vi "初始化.vi"(8 "error in (no error)":errorcluster caption="错误输入（无错误）", 11 "堆栈 输入":refnum<class "堆栈(STR).lvclass"> caption="DNL_LabVIEW Object in") -> (0 "error out":errorcluster caption="错误输出", 3 "堆栈输出":refnum<class "堆栈(STR).lvclass"> caption="DNL_LabVIEW Object out")   [LabVIEW 2012, in "堆栈(STR).lvclass"]
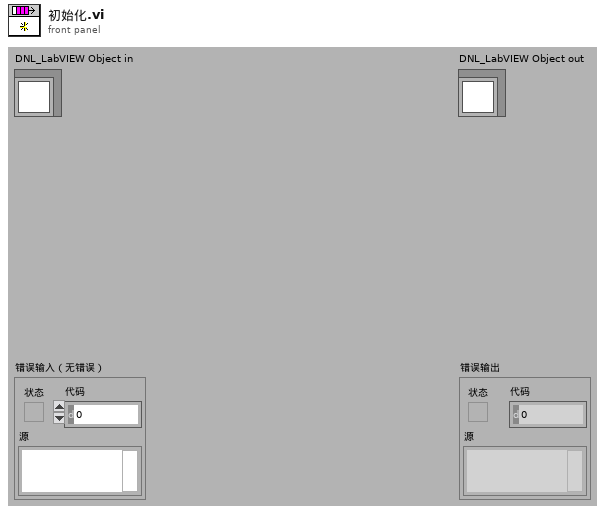
[diagram p1: front panel]
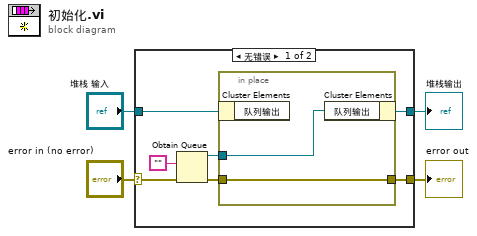
[diagram p0: block diagram]
diagram:
  n1 = case shown="无错误" "error in (no error)" {
    selector: "error in (no error)" -> [w8 w15]
    tunnel: [w6 w15] -> w3
    tunnel: [w9 w14] -> w1
    tunnel: "堆栈 输入" -> [w11 w14]
    frame No Error {
      n2 = Obtain Queue(element data type="", error in (no error)=w8) -> (queue out=w10:refnum<queue>, error out=w7:errorcluster)  [unwired: 3 in, 1 out]
      n3 = in-place {
        in-place-border: w10 -> [w13]
        in-place-border: w7 -> [w12]
        in-place-border: [w12] -> w6
        n4 = in-place-cluster #1(w11) -> ()  [unwired: 1 out]
        n5 = in-place-cluster #1("队列输出"=w13) -> (w9:refnum<class "堆栈(STR).lvclass">)
      }
    }
    frame Error {
    }
  }
  "error out" <- w3
  "堆栈输出" <- w1
